vi "HEWH Update Draw Amount Display.vi"(0 "Terminate Condition A":T1, 1 "Terminate Condition B":T1, 2 "Terminate Condition C":T1, 3 "Terminate Condition D":T1, 5 "Error In":errorcluster, 6 "Gallons to Draw A":dbl, 8 "Gallons to Draw B":dbl, 10 "Gallons to Draw C":dbl, 12 "Gallons to Draw D":dbl) -> (14 "Draw Amount (Station A)":dbl=15.0 caption="Draw Amount (Gal)", 15 "Draw Amount (Station B)":dbl=15.0 caption="Draw Amount (Gal)", 16 "Draw Amount (Station C)":dbl=15.0 caption="Draw Amount (Gal)", 17 "Draw Amount (Station D)":dbl=15.0 caption="Draw Amount (Gal)", 19 "Error Out":errorcluster)   [LabVIEW 2016]
uses:
  Draw Water Specific/Type Definitions/Terminate Draw Conditions.ctl
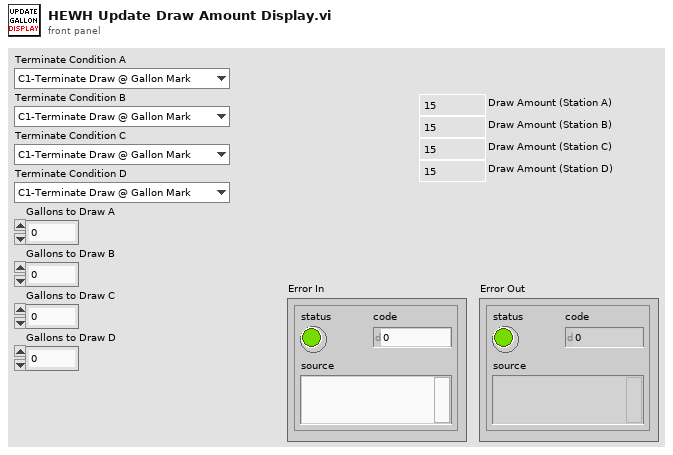
[diagram p1: front panel]
types:
  T1 = typedef "Terminate Draw Conditions.ctl" = enum16{"C1-Terminate Draw @ Gallon Mark", "C2-Special Last Draw (HU Test)", "C3-RTD Out <=", "C4-Mean Tank Temp <=", "C5-Decrease RTD Out (Deg F)", "C6-Time (Seconds)", "C7-Until Any Heat Source", "C8-Specific Heat Source", "C9-Do Nothing"}
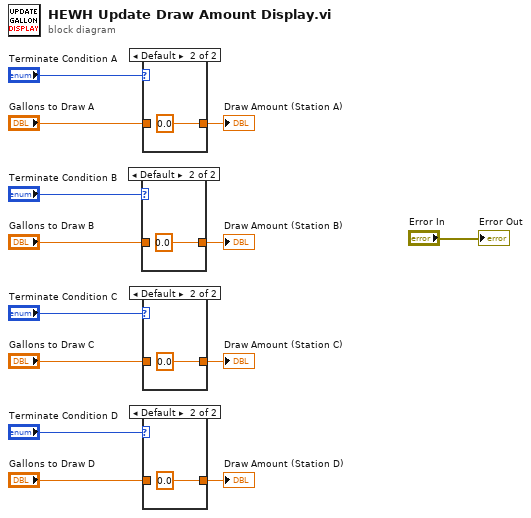
[diagram p0: block diagram]
diagram:
  n1 = case shown="Default" "Terminate Condition B" {
    tunnel: "Gallons to Draw B" -> [w14 _]
    tunnel: [w14 0.0 ("Gallons to Draw B")] -> w4
    frame "C1-Terminate Draw @ Gallon Mark" {
    }
    frame Default {
    }
  }
  "Draw Amount (Station B)" <- w4
  n2 = case shown="Default" "Terminate Condition A" {
    tunnel: "Gallons to Draw A" -> [w16 _]
    tunnel: [w16 0.0 ("Gallons to Draw A")] -> w5
    frame "C1-Terminate Draw @ Gallon Mark" {
    }
    frame Default {
    }
  }
  "Draw Amount (Station A)" <- w5
  n3 = case shown="Default" "Terminate Condition C" {
    tunnel: "Gallons to Draw C" -> [w18 _]
    tunnel: [w18 0.0 ("Gallons to Draw C")] -> w3
    frame "C1-Terminate Draw @ Gallon Mark" {
    }
    frame Default {
    }
  }
  "Draw Amount (Station C)" <- w3
  n4 = case shown="Default" "Terminate Condition D" {
    tunnel: "Gallons to Draw D" -> [w20 _]
    tunnel: [w20 0.0 ("Gallons to Draw D")] -> w2
    frame "C1-Terminate Draw @ Gallon Mark" {
    }
    frame Default {
    }
  }
  "Draw Amount (Station D)" <- w2
  "Error Out" <- "Error In"
